vi "Do.vi"(8 "error in (no error)":errorcluster, 10 "Actor in":refnum<class "Actor.lvclass">, 11 "Read Decimated Traces Msg":refnum<class "Read Decimated Traces Msg.lvclass">) -> (0 "error out":errorcluster, 2 "Actor out":refnum<class "Actor.lvclass">)   [LabVIEW 2017, in "BNT_DSCXtGraph.lvlib" / "Read Decimated Traces Msg.lvclass"]
doc: "This VI delivers the message to the actor by calling the appropriate method(s) on the actor."
uses:
  Read Decimated Traces Msg.lvclass
  <vilib>/ActorFramework/Actor/Actor.lvclass
  BNT_DSCXtGraph/BNT_DSCXtGraph.lvclass
  C:/Program Files (x86)/National Instruments/LabVIEW 2017/vi.lib/ActorFramework/Actor/Actor.lvclass
  CSPP_Core/Messages/CSPP_AsyncCallbackMsg/CSPP_AsyncCallback Msg.lvclass
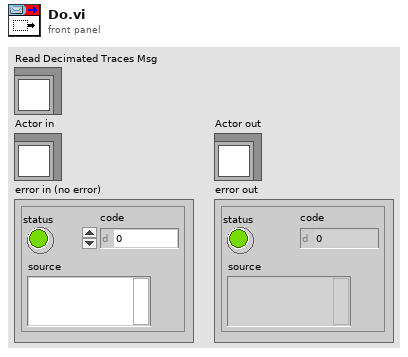
[diagram p1: front panel]
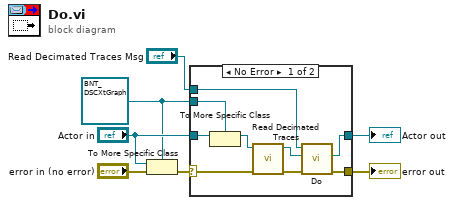
[diagram p0: block diagram]
diagram:
  w2 = refnum<class "BNT_DSCXtGraph.lvclass"> refnum ("Actor in")
  n1 = To More Specific Class(target class=w2, reference="Actor in", error in="error in (no error)") -> (error out=w6:errorcluster)  [unwired: 1 out]
  n2 = case shown="No Error" w6 {
    selector: w6 -> [w16 w18]
    tunnel: [w13 w18] -> w5
    tunnel: [w12 w17] -> w4
    tunnel: "Actor in" -> [w15 w17]
    tunnel: w2 -> [w14 _]
    tunnel: "Read Decimated Traces Msg" -> [w10 _]
    frame No Error {
      n3 = To More Specific Class ("To More Specific Class (internal)")(target class=w14, reference=w15) -> (specific class reference=w9:refnum<class "BNT_DSCXtGraph.lvclass">)  [unwired: 1 in, 1 out]
      n4 = call "Read Decimated Traces.vi"("Error In"=w16, "BNT_DSCXtGraph in"=w9) -> ("Error Out"=w11:errorcluster, "BNT_DSCXtGraph out"=w8:refnum<class "BNT_DSCXtGraph.lvclass">)  [unwired: 8 in]
      n5 = call-parent "Do.vi"("error in (no error)"=w11, "Actor in"=w8, "CSPP_AsyncCallback Msg"=w10) -> ("error out"=w13:errorcluster, "Actor out"=w12:refnum<class "Actor.lvclass">)  [unwired: 7 in]
    }
    frame Error {
    }
  }
  "error out" <- w5
  "Actor out" <- w4
